vi "mod_Costas loop.vi"(0 "extracted AM modulated signal":cluster{"t0":dbl, "dt":dbl, "Y":cdb[]}={"t0"=0.0, "dt"=1.0, "Y"=[]} {"Y" format="%.3f"; "dt" format="%^.2e"; "t0" format="%.4f"}, 5 "extracted pilot tone":cluster{"t0":dbl, "dt":dbl, "Y":cdb[]}={"t0"=0.0, "dt"=1.0, "Y"=[]} {"Y" format="%.3f"; "dt" format="%^.2e"; "t0" format="%.4f"}, 7 "pilot tone":dbl, 9 "costas loop parameters":T1={"Alpha"=0.001, "Beta"=2e-05} {"Beta" format="%#_6p"; "Alpha" format="%#_6p"}, 11 "error in (no error)":errorcluster, 13 "reset? (T)":bool=TRUE) -> (4 "recovered AM modulated signal":cluster{"t0":dbl, "dt":dbl, "Y":cdb[]}={"t0"=0.0, "dt"=1.0, "Y"=[]} {"Y" format="%.3f"; "dt" format="%^.2e"; "t0" format="%.4f"}, 6 "frequency offset":dbl, 8 "phase offset (degrees)":dbl, 15 "error out":errorcluster)   [LabVIEW 2020, in "niAMT.lvlib"]
uses:
  <vilib>/addons/Modulation/niAMT.lvlib
  <vilib>/addons/Modulation/Analog/controls/mod_Costas loop parameters.ctl
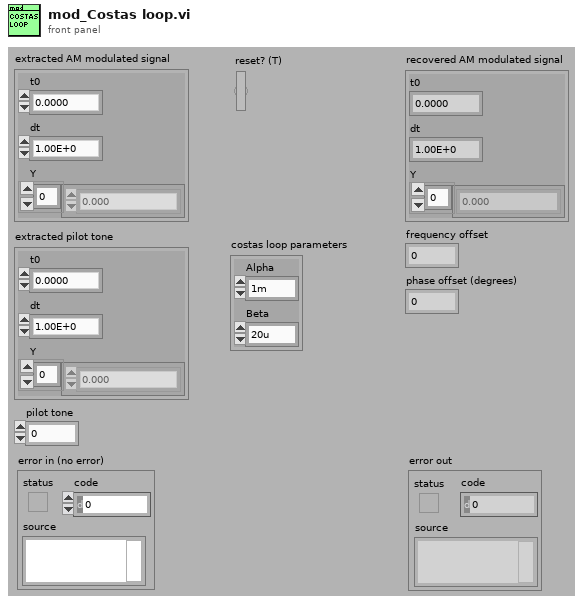
[diagram p1: front panel]
types:
  T1 = typedef "niAMT.lvlib/mod_Costas loop parameters.ctl" = cluster{"Alpha":dbl, "Beta":dbl}
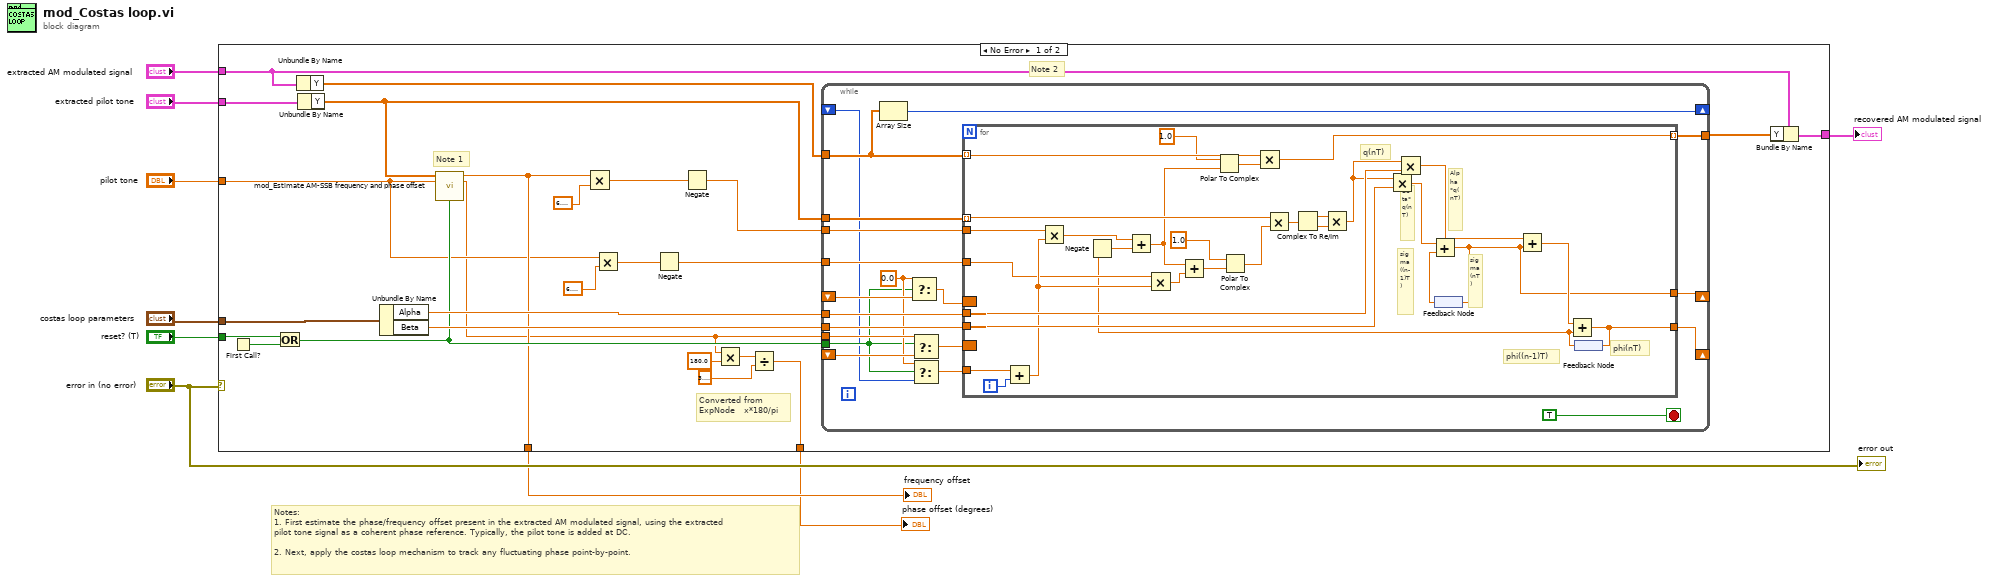
[diagram p0: block diagram]
diagram:
  # "Notes:\n1. First estimate the phase/frequency offset present in the extracted AM modulated signal, using the extracted\npilot tone signal as a coherent phase reference. Typically, the pilot tone is added at DC.\n\n2. Next, apply the costas loop mechanism to track any fluctuating phase point-by-point."
  n1 = case shown="No Error" "error in (no error)" {
    tunnel: [w16 _] -> w9
    tunnel: [w10 _] -> w1
    tunnel: "extracted AM modulated signal" -> [w17 _]
    tunnel: "extracted pilot tone" -> [w19 _]
    tunnel: "pilot tone" -> [w22 _]
    tunnel: "costas loop parameters" -> [w29 _]
    tunnel: "reset? (T)" -> [w28 _]
    tunnel: [w24 _] -> w2
    frame No Error {
      # "Converted from\nExpNode\t\t\tx*180/pi"
      # "Note 2"
      # "Note 1"
      n2 = First Call?() -> (First Call?: T/F=w32:bool)
      n3 = Or(x=w28, y=w32) -> (x .or. y?=w31:bool)
      n4 = Unbundle By Name(w17) -> ("Y"=w20:cdb[])
      n5 = Unbundle By Name(w19) -> ("Y"=w18:cdb[])
      n6 = Unbundle By Name(w29) -> ("Alpha"=w34:dbl, "Beta"=w33:dbl)
      n7 = call <vilib>:"mod_Estimate AM-SSB frequency and phase offset.vi"("extracted pilot tone signal"=w18, "pilot tone"=w22, "reset? (T)"=w31) -> ("frequency offset"=w24:dbl, "phase offset (radians)"=w11:dbl)  [unwired: 1 in, 10 out]
      n8 = Multiply(x=w24, y=6.283185307179586) -> (x*y=w27:dbl)
      n9 = Multiply(x=w22, y=6.283185307179586) -> (x*y=w23:dbl)
      n10 = Negate(x=w23) -> (-x=w26:dbl)
      n11 = Negate(x=w27) -> (-x=w25:dbl)
      n12 = Multiply(x=w11, y=180.0) -> (x*y=w13:dbl)
      n13 = Divide(x=w13, y=3.141592653589793) -> (x/y=w10:dbl)
      n14 = while {
        tunnel: w20 -> [w38]
        tunnel: w18 -> [w54]
        tunnel: w34 -> [w53]
        tunnel: w33 -> [w52]
        tunnel: w11 -> [w48]
        tunnel: [w51] -> w15
        tunnel: w31 -> [w37]
        shift-right: [w41] -> _
        shift-left: _ -> [w49]
        shift-right: [w42] -> _
        shift-left: _ -> [w44]
        tunnel: w25 -> [w40]
        tunnel: w26 -> [w39]
        shift-right: [w36] -> _
        shift-left: _ -> [w35]
        stop <- TRUE stop-if-true
        w43 = 0.0 ("t")
        n15 = Array Size(array=w38) -> (size(s)=w36:i32)
        n16 = Select(t=w43, s=w37, f=w44) -> (s? t:f=w45:dbl)
        n17 = Select(t=w48, s=w37, f=w49) -> (s? t:f=w46:dbl)
        n18 = Select(t=w43, s=w37, f=w35) -> (s? t:f=w47:dbl)
        n19 = for {
          tunnel: w38 -> [w69] mode=indexing
          tunnel: w54 -> [w82] mode=indexing
          tunnel: w53 -> [w78]
          tunnel: w52 -> [w76]
          tunnel: [w73] -> w51 mode=indexing
          tunnel: [w57] -> w42
          tunnel: w47 -> [w71]
          tunnel: [w68] -> w41
          tunnel: w40 -> [w67]
          tunnel: w39 -> [w63]
          border: w45 -> [_]
          border: w46 -> [_]
          i -> [w72]
          # "phi((n-1)T)"
          # "phi(nT)"
          # "sigma(nT)"
          # "Beta*q(nT)"
          # "sigma((n-1)T)"
          # "Alpha*q(nT)"
          # "q(nT)"
          n20 = Add(x=w71, y=w72) -> (x+y=w64:dbl)
          n21 = Multiply(x=w67, y=w64) -> (x*y=w84:dbl)
          n22 = Multiply(x=w63, y=w64) -> (x*y=w62:dbl)
          n23 = feedback #1() -> (w70:dbl)
          n24 = feedback #2() -> (w56:dbl)
          n25 = Negate(x=w56) -> (-x=w55:dbl)
          n26 = Add(x=w84, y=w55) -> (x+y=w59:dbl)
          n27 = Add(x=w59, y=w62) -> (x+y=w65:dbl)
          n28 = Polar To Complex(1:w59, 2:1.0) -> (0:w58:cdb)
          n29 = Polar To Complex(1:w65, 2:1.0) -> (0:w61:cdb)
          n30 = Multiply(x=w69, y=w58) -> (x*y=w73:cdb)
          n31 = Multiply(x=w82, y=w61) -> (x*y=w81:cdb)
          n32 = Complex To Re/Im(x + iy=w81) -> (x=w80:dbl, y=w79:dbl)
          n33 = Multiply(x=w80, y=w79) -> (x*y=w74:dbl)
          n34 = Multiply(x=w74, y=w76) -> (x*y=w75:dbl)
          n35 = Multiply(x=w74, y=w78) -> (x*y=w77:dbl)
          n36 = Add(x=w75, y=w70) -> (x+y=w57:dbl)
          n37 = feedback-in #1(w57) -> ()
          n38 = Add(x=w77, y=w57) -> (x+y=w66:dbl)
          n39 = Add(x=w66, y=w56) -> (x+y=w68:dbl)
          n40 = feedback-in #2(w68) -> ()
        }
      }
      n41 = Bundle By Name(cluster=w17, "Y"=w15) -> (w16:cluster{"t0":dbl, "dt":dbl, "Y":cdb[]})
    }
    frame Error {
    }
  }
  "recovered AM modulated signal" <- w9
  "frequency offset" <- w2
  "phase offset (degrees)" <- w1
  "error out" <- "error in (no error)"
